vi "DequeueMainController.vi"(8 "error in (no error)":errorcluster, 10 "timeout in ms (-1)":i32=-1, 11 "MainQueue":refnum<queue>) -> (0 "error out":errorcluster, 1 "Data":variant, 2 "Message":T1=enum."Exit", 3 "MainQueue out":refnum<queue>, 4 "timed out?":bool)   [LabVIEW 2019, in "MainController.lvlib"]
uses:
  MainController.lvlib
  Cluster - MainControllerMessage.ctl
  Enum - MainState.ctl
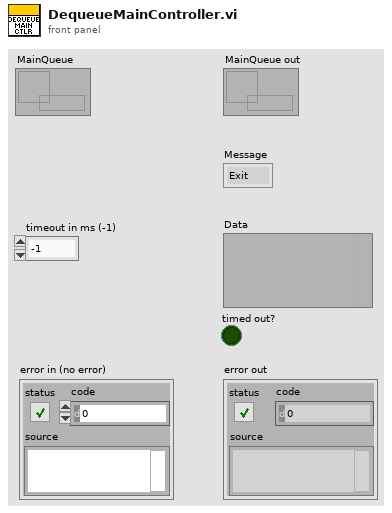
[diagram p1: front panel]
types:
  T1 = typedef "MainController.lvlib/Enum - MainState.ctl" = enum16{"Initialize", "InitUIRefs", "LaunchSettings", "LaunchAutoMode", "LaunchManualMode", "LaunchTestReport", "ConnectHardware", "DisconnectHardware", "HiliteNavItems", "StartAutoMode", "PauseAutoMode", "StopAutoMode", "ShowFlyout", "HideFlyout", "BroadcastSettings", "PickupTestSettings", "BroadcastHW", "AutoTestDone", "DAQStatus", "UpdateCommandBar", "Error", "RecieveError", "Exit"}
  T2 = typedef "MainController.lvlib/Cluster - MainControllerMessage.ctl" = cluster{"Message":T1, "Data":variant}
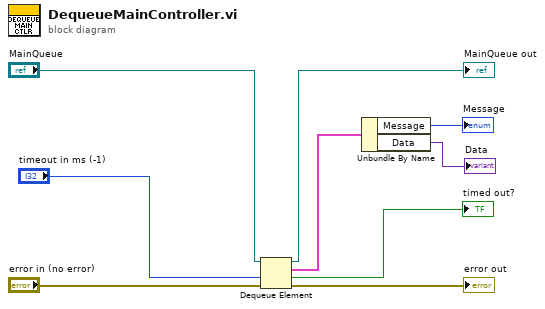
[diagram p0: block diagram]
diagram:
  n1 = Dequeue Element(queue="MainQueue", timeout in ms (-1)="timeout in ms (-1)", error in (no error)="error in (no error)") -> (queue out=→"MainQueue out":refnum<queue>, element=w3:T2, timed out?=→"timed out?":bool, error out=→"error out":errorcluster)
  n2 = Unbundle By Name(w3) -> ("Message"=→"Message":T1, "Data"=→"Data":variant)
